vi "TEST_L1_ADDER_TEST.vi"(5 "Serial Number":string="SN_00327", 6 "error in":errorcluster, 9 "Instrument VISA in":T1={"AWG VISA"="AgilentGenerator1", "Oscilloscope  VISA "="AgilentOsciloscope", "Integration Board IP"="172.16.17.48", "connection ID"=refnum, "report out"=refnum, "report file path"=path "C:/Users/omartinez/Desktop/L0nL1_Results"}) -> (0 "error out":errorcluster, 3 "VISA Out":T1={"AWG VISA"="AgilentGenerator1", "Oscilloscope  VISA "="AgilentOsciloscope", "Integration Board IP"="172.16.17.48", "connection ID"=refnum, "report out"=refnum, "report file path"=path "C:/Users/omartinez/Desktop/L0nL1_Results"})   [LabVIEW 2012]
uses:
  <vilib>/Utility/NIReport.llb/NI_report.lvclass
  <vilib>/Utility/NIReport.llb/HTML/NI_HTML.lvclass
  <instrlib>/Agilent 8000 Series/Agilent 8000 Series.lvlib
  Sum_Abrilader/L0_Sum_Adder Folder/C/Program Files/National Instruments/LabVIEW 2012/instr.lib/Agilent 81150/Agilent 81150.lvlib
panel:
  in  "Modes REG100&101 Values":u32[][](array[numeric])=[[45565, 1022], [42239, 1022], [32925, 1020]]
  in  "Threshold Limits":i16[](array[numeric])=[0, 512]
  out "Threshold\nLimits":u16[](array[numeric])=[98, 99]
  in  "Pulse Amplitudes":dbl[](array[numeric])=[0.4]
  in  "Combination\n  (Act High)":i32 min=0 max=127 step=1 format="%b"
  in  "Single/Comb":bool
  in  "Single Channel Enable":i32(slide) scale=0.0..6.0
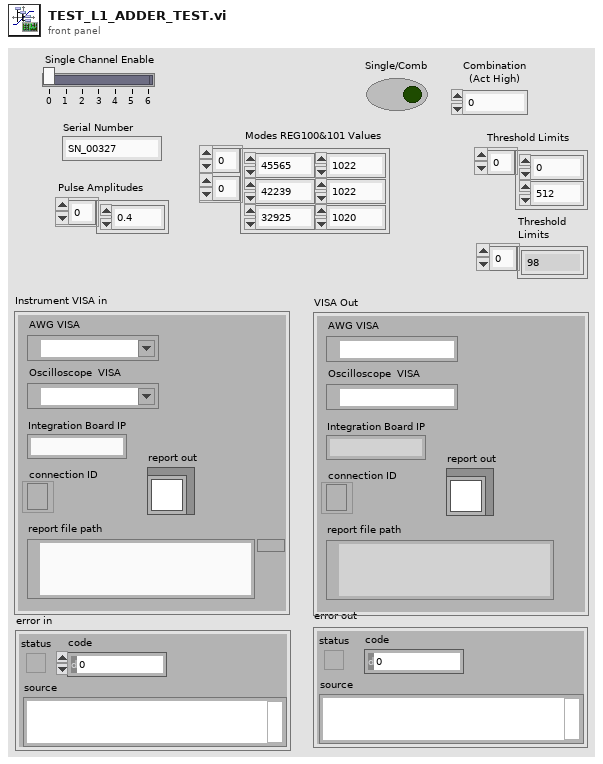
[diagram p1: front panel]
types:
  T1 = cluster{"AWG VISA":refnum<visa-resource-name>, "Oscilloscope  VISA ":refnum<visa-resource-name>, "Integration Board IP":string, "connection ID":refnum<k5>, "report out":refnum<class "NI_report.lvclass">, "report file path":path}
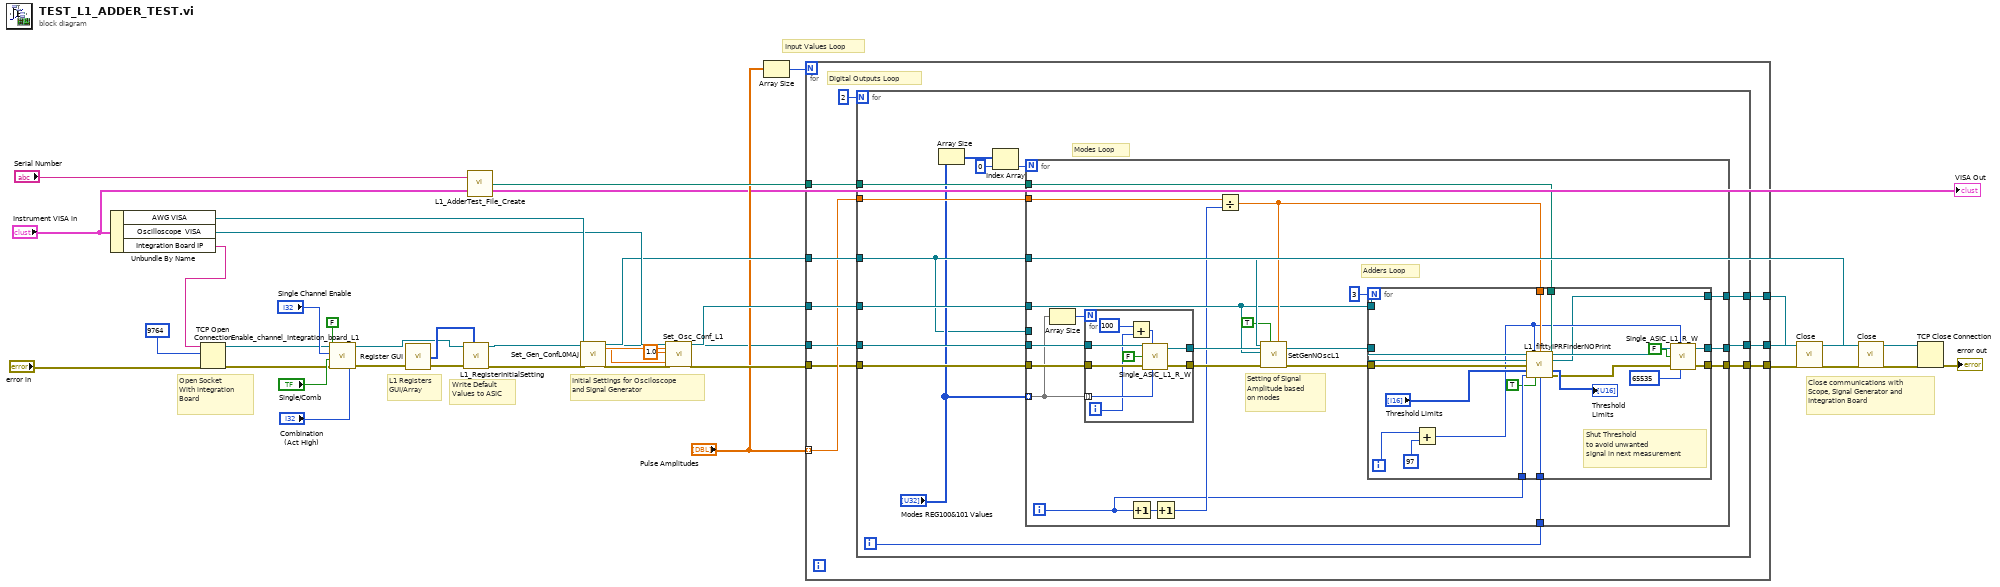
[diagram p0: block diagram]
diagram:
  # "Input Values Loop"
  # "Write Default\nValues to ASIC"
  # "Close communications with \nScope, Signal Generator and \nIntegration Board"
  # "Initial Settings for Osciloscope\nand Signal Generator"
  # "L1 Registers\nGUI/Array"
  # "Open Socket\nWith integration \nBoard"
  n1 = Unbundle By Name("Instrument VISA in") -> ("AWG VISA"=w23:refnum<visa-resource-name>, "Oscilloscope  VISA"=w22:refnum<visa-resource-name>, "Integration Board IP"=w28:string)
  n2 = TCP Open Connection(address=w28, remote port or service name=9764, error in (no error)="error in") -> (connection ID=w10:refnum<k5>, error out=w1:errorcluster)  [unwired: 2 in]
  n3 = call "Enable_channel_Integration_board_L1.vi"("Combination"="Combination\n  (Act High)", "Enable  L1 single  Input"="Single Channel Enable", "error in (no error)"=w1, "SingleIN/#Combination"="Single/Comb", "Enable some/all"=FALSE ("#Enable all L1"), "connection ID"=w10) -> ("error out"=w2:errorcluster, "connection ID out"=w3:refnum<k5>)
  n4 = call "Register GUI.vi"("error in (no error)"=w2) -> ("error out"=w4:errorcluster, "REG ARRAy"=w5:u32[])  [unwired: 3 in]
  n5 = call "L1_RegisterInitialSetting.vi"("REG ARRAy"=w5, "error in"=w4, "connection ID in"=w3) -> ("error out"=w7:errorcluster, "connection ID out"=w6:refnum<k5>)  [unwired: 7 in]
  n6 = call "L1_AdderTest_File_Create.vi"("input cluster"="Instrument VISA in", "Serial Number"="Serial Number") -> ("appended path"=w27:path)
  n7 = call "Set_Gen_ConfL0MAJ.vi"("AWG VISA"=w23, "error in (no error)"=w7) -> ("Amplitude 1 OUT"=w25:dbl, "VISA resource name out"=w14:refnum<visa-resource-name>, "Pulse Width in seconds 1 OUT"=w24:dbl, "error out"=w26:errorcluster)  [unwired: 10 in, 4 out]
  n8 = call "Set_Osc_Conf_L1.vi"("VISA resource name"=w22, "Amplitude IN"=w25, "Trigger Level IN"=1.0, "Pulse Width in seconds IN"=w24, "error in (no error)"=w26) -> ("VISA resource name out"=w16:refnum<visa-resource-name>, "error out"=w17:errorcluster)  [unwired: 13 in]
  n9 = Array Size(array="Pulse Amplitudes") -> (size(s)=w13:i32)
  n10 = for {
    N: w13 -> [_]
    tunnel: [w45] -> w29
    tunnel: w27 -> [w44]
    tunnel: w6 -> [w43]
    tunnel: [w42] -> w21
    tunnel: [w41] -> w18
    tunnel: w17 -> [w36]
    tunnel: w16 -> [w40]
    tunnel: w14 -> [w39]
    tunnel: "Pulse Amplitudes" -> [w38] mode=indexing
    # "Digital Outputs Loop"
    n11 = for {
      N: 2 -> [_]
      tunnel: [w59] -> w45
      tunnel: w44 -> [w58]
      tunnel: w43 -> [w57]
      tunnel: [w56] -> w42
      tunnel: [w55] -> w41
      tunnel: w36 -> [w54]
      tunnel: w40 -> [w53]
      tunnel: w39 -> [w46]
      tunnel: w38 -> [w52]
      i -> [w47]
      # "Modes Loop"
      n12 = Array Size(array="Modes REG100&101 Values") -> (size(s)=w51:i32[])
      n13 = Index Array(array=w51, index=0) -> (element=w50:i32)
      n14 = for {
        N: w50 -> [_]
        tunnel: [w80] -> w56
        tunnel: [w78] -> w59
        tunnel: w57 -> [w73]
        tunnel: w58 -> [w77]
        tunnel: w52 -> [w75]
        tunnel: w54 -> [w74]
        tunnel: w53 -> [w64]
        tunnel: [w76] -> w55
        tunnel: w46 -> [_]
        tunnel: "Modes REG100&101 Values" -> [w71] mode=indexing
        tunnel: w47 -> [w69]
        tunnel: w46 -> [w65]
        i -> [w60]
        # "Setting of Signal\nAmplitude based \non modes"
        # "Adders Loop"
        n15 = Array Size(array=w71) -> (size(s)=w70:i32)
        n16 = for {
          N: w70 -> [_]
          tunnel: w74 -> [w89]
          tunnel: [w88] -> w67
          tunnel: w73 -> [w87]
          tunnel: [w86] -> w72
          tunnel: w71 -> [w85] mode=indexing
          i -> [w83]
          n17 = Add(x=100, y=w83) -> (x+y=w84:i32)
          n18 = call "Single_ASIC_L1_R_W.vi"("connection ID"=w87, "Register or channel"=w84, "RD/#WR"=FALSE, "error in (no error)"=w89, "Data"=w85) -> ("connection ID out"=w86:refnum<k5>, "error out"=w88:errorcluster)  [unwired: 1 in, 2 out]
        }
        n19 = Increment(x=w60) -> (x+1=w62:i32)
        n20 = Increment(x=w62) -> (x+1=w61:i32)
        n21 = Divide(x=w75, y=w61) -> (x/y=w66:dbl)
        n22 = call "SetGenNOscL1.vi"("Input Voltage"=w66, "Enable Output"=TRUE, "error in (no error)"=w67, "VISA resource name"=w64, "AWG VISA"=w65) -> ("error out 2"=w68:errorcluster)  [unwired: 6 in]
        n23 = for {
          N: 3 -> [_]
          tunnel: w72 -> [w99]
          tunnel: w68 -> [w100]
          tunnel: [w107] -> w80
          tunnel: [w106] -> w78
          tunnel: w77 -> [w102]
          tunnel: w66 -> [w103]
          tunnel: w64 -> [w101]
          tunnel: [w93] -> w76
          tunnel: w69 -> [w92]
          tunnel: w60 -> [w91]
          i -> [w108]
          # "Shut Threshold\nto avoid unwanted\nsignal in next measurement"
          n24 = Add(x=w108, y=97) -> (x+y=w97:i32)
          n25 = call "L1_fifttyIPRFinderNOPrint.vi"("VISA In"=w101, "Adder Register"=w97, "Vin"=w103, "File path In"=w102, "ID In"=w99, "Error In"=w100, "Threshold Limits In"="Threshold Limits", "Channel/Mode"=w91, "Adder Test?"=TRUE, "Digital Output"=w92) -> ("ID out"=w94:refnum<k5>, "VISA Out"=w93:refnum<visa-resource-name>, "Threshold Limits Out"=→"Threshold\nLimits":i16[], "Error Out"=w95:errorcluster)  [unwired: 2 in]
          n26 = call "Single_ASIC_L1_R_W.vi"("connection ID"=w94, "Register or channel"=w97, "RD/#WR"=FALSE, "error in (no error)"=w95, "Data"=u32 65535 ("COMB DEC")) -> ("connection ID out"=w106:refnum<k5>, "error out"=w107:errorcluster)  [unwired: 1 in, 2 out]
        }
      }
    }
  }
  n27 = call <instrlib>:"Close.vi"("error in (no error)"=w21, "VISA resource name"=w18) -> ("error out"=w20:errorcluster)  [unwired: 9 in]
  n28 = call <instrlib>:"Close.vi"("error in (no error)"=w20, "VISA resource name"=w14) -> ("error out"=w19:errorcluster)  [unwired: 9 in]
  n29 = TCP Close Connection(connection ID=w29, error in (no error)=w19) -> (error out=→"error out":errorcluster)  [unwired: 1 in, 1 out]
  "VISA Out" <- "Instrument VISA in"
